vi "Demo - Sort text.vi"() -> ()   [LabVIEW 2014]
uses:
  HMM.lvlib
panel:
  out "Estimated HMM":T1
  out "Iteration":i32
  out "Estimated b":dbl[][](graph)
  out "Probability(LOG)":dbl(graph)
  in  "#iterations":i32=1000
  out "Initial b":dbl[][](graph)
  out "Initial HMM":T1
  in  "M #observed states":i32=27
  in  "N #hidden states":i32=2
  out "size(s)":i32
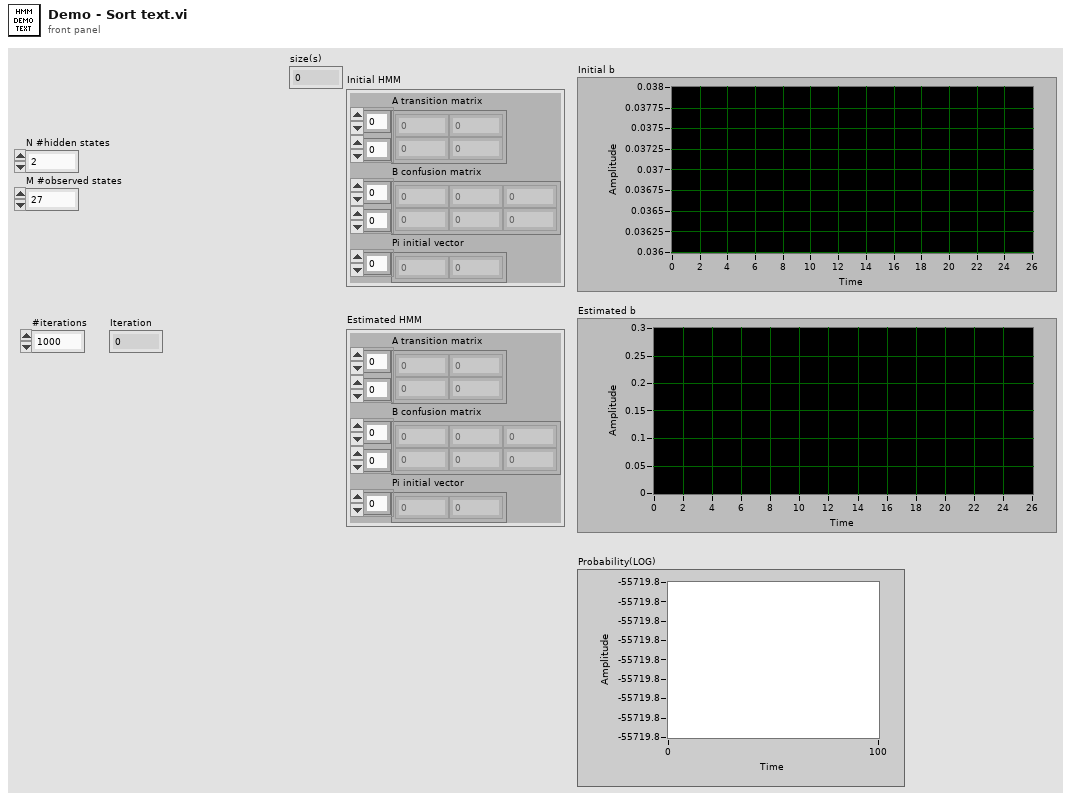
[diagram p1: front panel]
types:
  T1 = cluster{"A transition matrix":dbl[][], "B confusion matrix":dbl[][], "Pi initial vector":dbl[]}
  T2 = typedef "HMM.lvlib/HMM Cluster.ctl" = cluster{"A transition matrix":dbl[][], "B confusion matrix":dbl[][], "Pi initial vector":dbl[]}
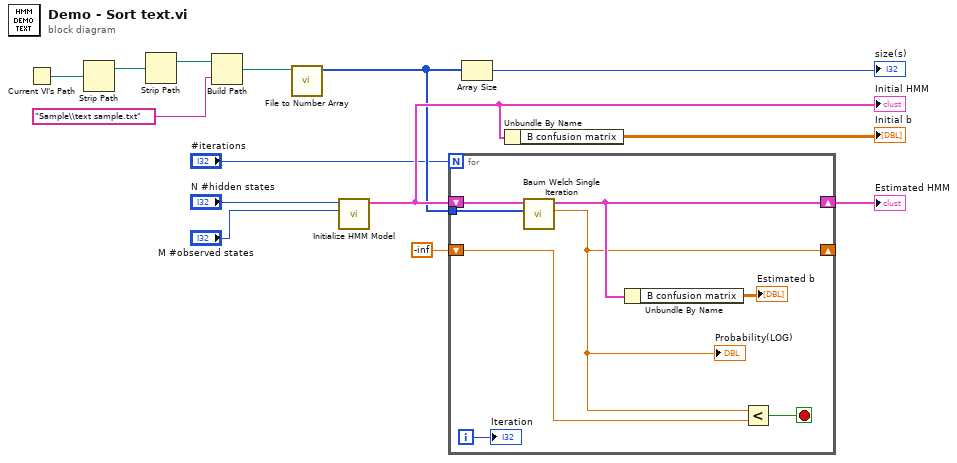
[diagram p0: block diagram]
diagram:
  n1 = Current VI's Path() -> (path=w5:path)
  n2 = Strip Path(path=w5) -> (stripped path=w4:path)  [unwired: 1 out]
  n3 = Strip Path(path=w4) -> (stripped path=w3:path)  [unwired: 1 out]
  n4 = Build Path(base path=w3, name or relative path="Sample\\text sample.txt") -> (appended path=w1:path)
  n5 = call "File to Number Array.vi"("file path"=w1) -> ("Array"=w9:i32[])  [unwired: 8 in, 2 out]
  n6 = call "Initialize HMM Model.vi"("M #observed states"="M #observed states", "N #hidden states"="N #hidden states") -> ("Init HMM"=w10:T2)  [unwired: 9 in]
  "Initial HMM" <- w10
  n7 = for {
    N: "#iterations" -> [_]
    tunnel: w9 -> [w21]
    shift-right: [w16] -> _
    shift-left: -inf -> [w20]
    shift-right: [w17] -> w6
    shift-left: w10 -> [w22]
    i -> [w15]
    stop <- w19 stop-if-true
    n8 = call "Baum Welch Single Iteration.vi"("Observed states"=w21, "Init HMM"=w22) -> ("Log10(Prob)"=w16:dbl, "Estimated HMM"=w17:T2)  [unwired: 8 in]
    "Probability(LOG)" <- w16
    n9 = Unbundle By Name(w17) -> ("B confusion matrix"=→"Estimated b":dbl[][])
    n10 = Less?(x=w16, y=w20) -> (x < y?=w19:bool)
    "Iteration" <- w15
  }
  "Estimated HMM" <- w6
  n11 = Array Size(array=w9) -> (size(s)=→"size(s)":i32)
  n12 = Unbundle By Name(w10) -> ("B confusion matrix"=→"Initial b":dbl[][])
